vi "Export_Set Export File Setting.vi"(11 "Export Setting in":T1) -> (3 "Export Setting out":T1)   [LabVIEW 2015, in "ConfigHelper.lvlib"]
uses:
  ConfigHelper.lvlib
  Control_UI_Export Setting.ctl
  Control_UI_Export Setting State.ctl
  <vilib>/addons/PointValueMap/controls/PointMap.ctl
  Control_Export File Setup.ctl
  <vilib>/addons/PointValueMap/PointValueMap.lvlib
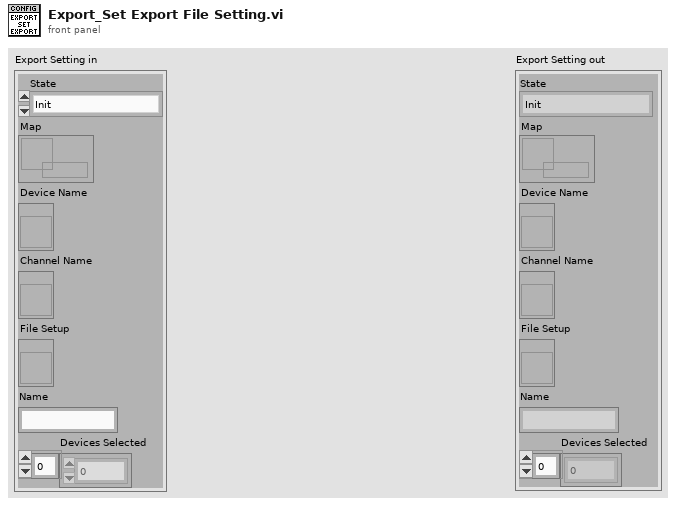
[diagram p1: front panel]
types:
  T1 = typedef "ConfigHelper.lvlib/Control_UI_Export Setting.ctl" = cluster{"State":T2, "Map":T3, "Device Name":refnum<vi>, "Channel Name":refnum<vi>, "File Setup":refnum<vi>, "Name":string, "Devices Selected":i32[]}
  T2 = typedef "ConfigHelper.lvlib/Control_UI_Export Setting State.ctl" = enum16{"Init", "Wait", "Exit", "Write to File", "Read from PVM", "Write to PVM", "Update Device", "Add Device", "Remove Device", "Copy Device", "Update Channel", "Add Channel", "Remove Channel", "Import from TDMS"}
  T3 = typedef "PointValueMap.lvlib/PointMap.ctl" = refnum<data-value>
  T4 = typedef "ConfigHelper.lvlib/Control_Export File Setup.ctl" = cluster{"CSV":bool, "TDMS":bool, "RAW TDMS":bool}
  T5 = typedef "ConfigHelper.lvlib/Control_Export Setup.ctl" = cluster{"Device Name":string, "Export CSV":bool, "Export TDMS":bool, "Export RAW TDMS":bool, "Channel Names":string[]}
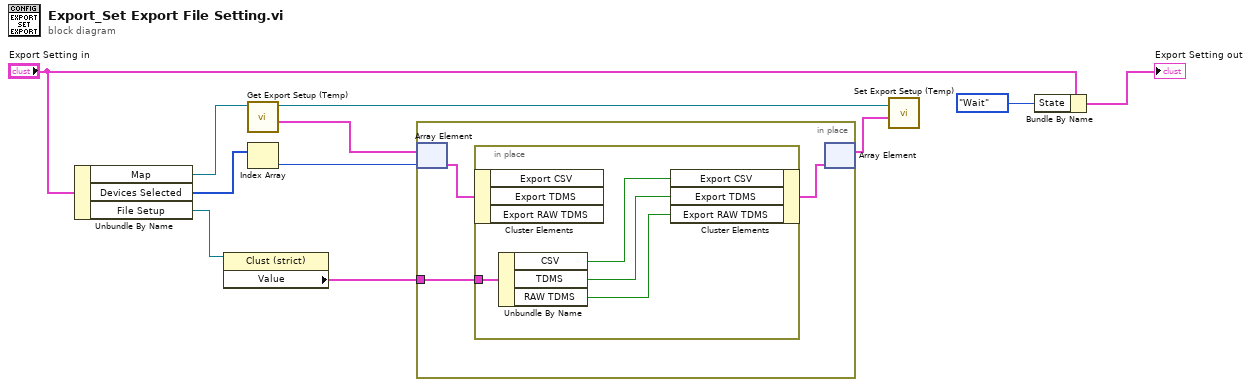
[diagram p0: block diagram]
diagram:
  n1 = Unbundle By Name("Export Setting in") -> ("Map"=w7:T3, "Devices Selected"=w5:i32[], "File Setup"=w8:refnum<vi>)
  n2 = property class="Clust (strict)"(reference=w8) -> ("Value"=w3:T4)  [unwired: 1 in, 2 out]
  n3 = call "Get Export Setup (Temp).vi"("Map"=w7) -> ("Export Setup"=w6:T5[], "Map Out"=w2:T3)  [unwired: 8 in, 1 out]
  n4 = Index Array(array=w5) -> (element=w4:i32)  [unwired: 1 in]
  n5 = in-place {
    in-place-border: w3 -> [w13]
    n6 = in-place-array #1(w6, w4) -> (w14:T5)
    n7 = in-place {
      in-place-border: w13 -> [w18]
      n8 = in-place-cluster #2(w14) -> ()  [unwired: 3 out]
      n9 = Unbundle By Name(w18) -> ("CSV"=w17:bool, "TDMS"=w16:bool, "RAW TDMS"=w15:bool)
      n10 = in-place-cluster #2("Export CSV"=w17, "Export TDMS"=w16, "Export RAW TDMS"=w15) -> (w12:T5)
    }
    n11 = in-place-array #1(w12) -> (w1:T5[])  [unwired: 1 out]
  }
  n12 = call "Set Export Setup (Temp).vi"("Export Setup"=w1, "Map"=w2) -> ()  [unwired: 8 in, 2 out]
  n13 = Bundle By Name(cluster="Export Setting in", "State"=Control_UI_Export_Setting_State."Wait") -> (→"Export Setting out":T1)
